vi "Construct New Connection Policy.vi"(11 "Return Queue":refnum<class "Message Enqueuer.lvclass">) -> (3 "New Connection Policy out":refnum<class "New Connection Policy.lvclass">)   [LabVIEW 2019, in "PersitantConnectionHandler.lvlib" / "New Connection Policy.lvclass"]
uses:
  <vilib>/gpm_packages/@cs/Network-interface/Source/PersistantConnectionHandler/New Connection Policy/New Connection Policy.lvclass
  <vilib>/ActorFramework/Message Enqueuer/Message Enqueuer.lvclass
  <vilib>/gpm_packages/@cs/Network-interface/Source/PersistantConnectionHandler/New Connection Policy/New Connection Policy.lvclass/New Connection Policy.ctl
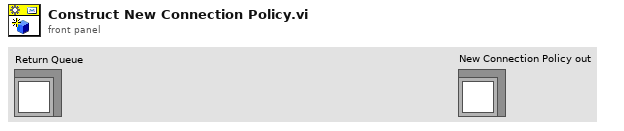
[diagram p1: front panel]
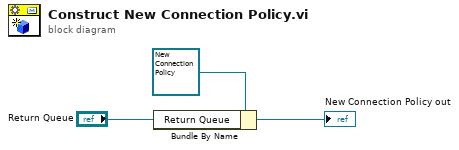
[diagram p0: block diagram]
diagram:
  n1 = Bundle By Name(cluster=refnum<class "New Connection Policy.lvclass"> refnum ("New Connection Policy in"), "Return Queue"="Return Queue") -> (→"New Connection Policy out":refnum<class "New Connection Policy.lvclass">)
